vi "Hi-Tec_conversions.vi"(0 "Input":dbl format="%.3f", 1 "Conversion":T2(ring), 2 "Release temp (deg C)":dbl format="%.2f", 3 "Atmos Pres (mbars)":dbl format="%.2f", 4 "Hi-Tec calib":T1={"Ref temp (deg C)"=0.0, "Ref Pres (mbars)"=0.0, "Density at calib conditions"=-0.0141, "Coefficients"=[]} {"Coefficients" format="%.2f"; "Density at calib conditions" format="%.4f"; "Ref Pres (mbars)" format="%.2f"; "Ref temp (deg C)" format="%.2f"}) -> (6 "Output":dbl format="%.3f", 7 "Flowrate (kg/min)":dbl format="%.4f")   [LabVIEW 2010]
uses:
  Controls/Hi-Tec_calib.ctl
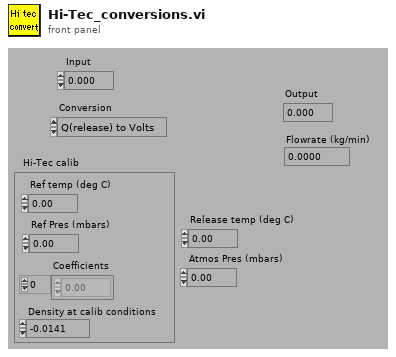
[diagram p1: front panel]
types:
  T1 = typedef "Hi-Tec_calib.ctl" = cluster{"Ref temp (deg C)":dbl, "Ref Pres (mbars)":dbl, "Density at calib conditions":dbl, "Coefficients":dbl[]}
  T2 = enum16{"Q(release) to Volts", "Volts to Q(release)"}
  T3 = enum16{"Release to Reference", "Reference to Release"}
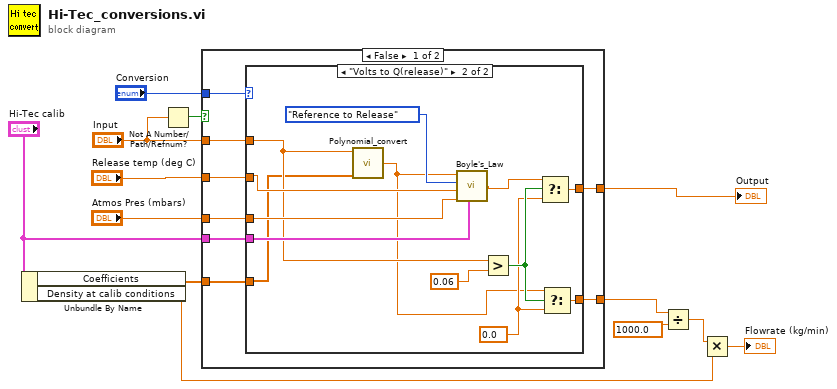
[diagram p0: block diagram]
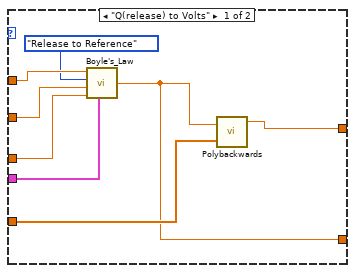
[diagram p2: hidden frame]
diagram:
  n1 = Unbundle By Name("Hi-Tec calib") -> ("Coefficients"=w12:dbl[], "Density at calib conditions"=w5:dbl)
  n2 = Not A Number/Path/Refnum?(number/path/refnum="Input") -> (NaN/Path/Refnum?=w1:bool)
  n3 = case shown="False" w1 {
    tunnel: "Conversion" -> [w21 _]
    tunnel: "Input" -> [w20 w43]
    tunnel: w12 -> [w19 _]
    tunnel: [w18 w43] -> w11
    tunnel: "Release temp (deg C)" -> [w17 _]
    tunnel: "Atmos Pres (mbars)" -> [w16 _]
    tunnel: "Hi-Tec calib" -> [w15 _]
    tunnel: [w14 w43] -> w3
    frame False {
      n4 = case shown="\"Volts to Q(release)\"" w21 {
        tunnel: w20 -> [w29 w32]
        tunnel: w19 -> [w24 w31]
        tunnel: [w22 w37] -> w18
        tunnel: w17 -> [w27 w40]
        tunnel: w16 -> [w26 w39]
        tunnel: w15 -> [w25 w41]
        tunnel: [w23 w35] -> w14
        frame "Q(release) to Volts" {
          n5 = call "Boyle's_Law.vi"("Q in (l/min)"=w29, "Conversion"=T3."Release to Reference", "Release temp (deg C)"=w27, "Atmos Pres (mbars)"=w26, "Hi-Tec calib"=w25) -> ("Q out (l/min)"=w23:dbl)  [unwired: 2 out]
          n6 = call "Polybackwards.vi"("Coefficients"=w24, "Y input"=w23) -> ("X output"=w22:dbl)  [unwired: 1 out]
        }
        frame "Volts to Q(release)" {
          w34 = 0.0 ("f")
          n7 = call "Polynomial_convert.vi"("Calib constants"=w31, "Voltage"=w32) -> ("Eng Values"=w30:dbl)  [unwired: 4 out]
          n8 = call "Boyle's_Law.vi"("Q in (l/min)"=w30, "Conversion"=T3."Reference to Release", "Release temp (deg C)"=w40, "Atmos Pres (mbars)"=w39, "Hi-Tec calib"=w41) -> ("Q out (l/min)"=w38:dbl)  [unwired: 2 out]
          n9 = Greater?(x=w32, y=0.06) -> (0:w36:bool)
          n10 = Select(t=w38, s=w36, f=w34) -> (s? t:f=w37:dbl)
          n11 = Select(t=w30, s=w36, f=w34) -> (s? t:f=w35:dbl)
        }
      }
    }
    frame True {
    }
  }
  "Output" <- w11
  n12 = Divide(x=w3, y=1000.0) -> (x/y=w6:dbl)
  n13 = Multiply(x=w6, y=w5) -> (x*y=→"Flowrate (kg/min)":dbl)
